vi "Generate Executed Tests Fraction String.vi"(8 "error in (no error)":errorcluster, 11 "Coverage Analyzer Result View in":refnum<class "Coverage Analyzer Result View.lvclass">) -> (0 "error out":errorcluster, 2 "Fraction of VIs Executed":string, 3 "Coverage Analyzer Result View out":refnum<class "Coverage Analyzer Result View.lvclass">)   [LabVIEW 2020, in "Coverage Analyzer Result View.lvclass"]
uses:
  Coverage Analyzer Result View.lvclass
  Coverage Analyzer Result View.lvclass/Coverage Analyzer Result View.ctl
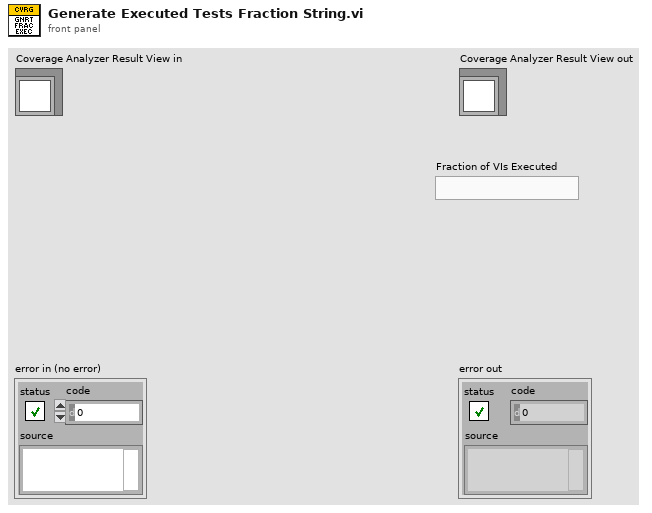
[diagram p1: front panel]
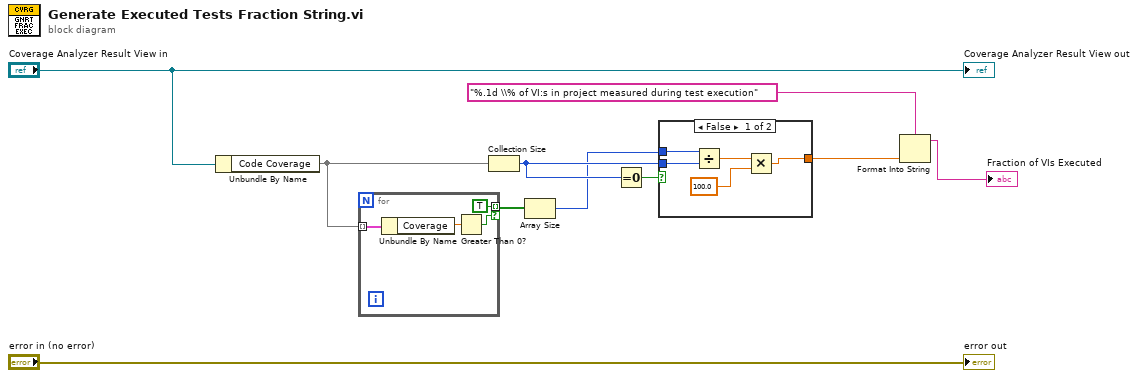
[diagram p0: block diagram]
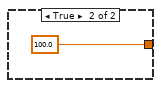
[diagram p2: hidden frame]
diagram:
  n1 = Unbundle By Name("Coverage Analyzer Result View in") -> ("Code Coverage"=w2:map{path, dbl})
  n2 = for {
    tunnel: w2 -> [w14] mode=indexing
    tunnel: [TRUE] -> w3 mode=indexing if=w11
    n3 = Unbundle By Name(w14) -> ("Coverage"=w13:dbl)
    n4 = Greater Than 0?(x=w13) -> (x > 0?=w11:bool)
  }
  n5 = Collection Size(1:w2) -> (0:w5:i32)
  n6 = Array Size(array=w3) -> (size(s)=w1:i32)
  n7 = Equal To 0?(x=w5) -> (x = 0?=w6:bool)
  n8 = case shown="False" w6 {
    tunnel: w1 -> [w19 _]
    tunnel: [w16 100.0] -> w4
    tunnel: w5 -> [w17 _]
    frame False {
      n9 = Divide(x=w19, y=w17) -> (x/y=w18:dbl)
      n10 = Multiply(x=w18, y=100.0) -> (x*y=w16:dbl)
    }
    frame True {
    }
  }
  n11 = Format Into String(format string="%.1d \\% of VI:s in project measured during test execution", w4) -> (resulting string=→"Fraction of VIs Executed":string)  [unwired: 2 in, 1 out]
  "error out" <- "error in (no error)"
  "Coverage Analyzer Result View out" <- "Coverage Analyzer Result View in"
